vi "instance count allowed.vi"(8 "error in":errorcluster, 11 "tag select module configuration in":refnum<class "Table Test configuration.lvclass">) -> (0 "error out":errorcluster, 2 "instances allowed":i32, 3 "tag select module configuration out":refnum<class "Table Test configuration.lvclass">)   [LabVIEW 2013, in "Table Test configuration.lvclass"]
uses:
  Table Test configuration.lvclass
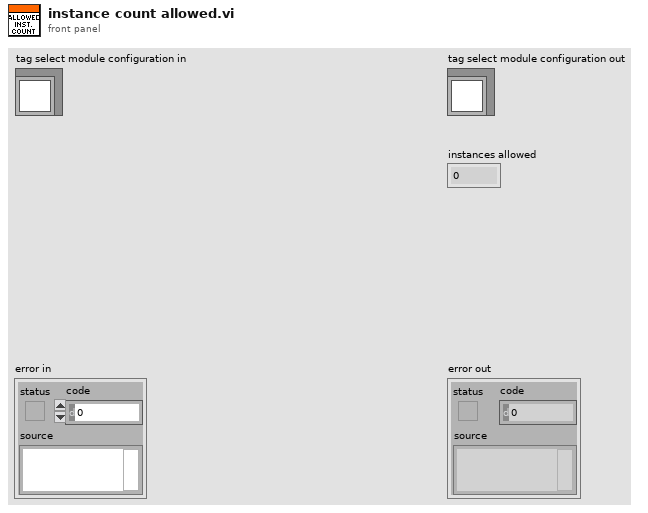
[diagram p1: front panel]
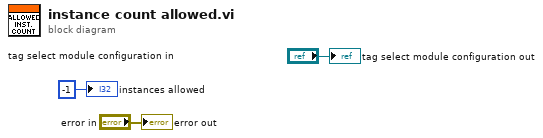
[diagram p0: block diagram]
diagram:
  "error out" <- "error in"
  "tag select module configuration out" <- "tag select module configuration in"
  "instances allowed" <- -1 ("instances allowed")
